vi "LocalisationFileLoader.vi"(11 "FilePath":path) -> (3 "LocalisationFileContent[out]":T1)   [LabVIEW 2012]
uses:
  <vilib>/Utility/file.llb/Read From Spreadsheet File (string).vi
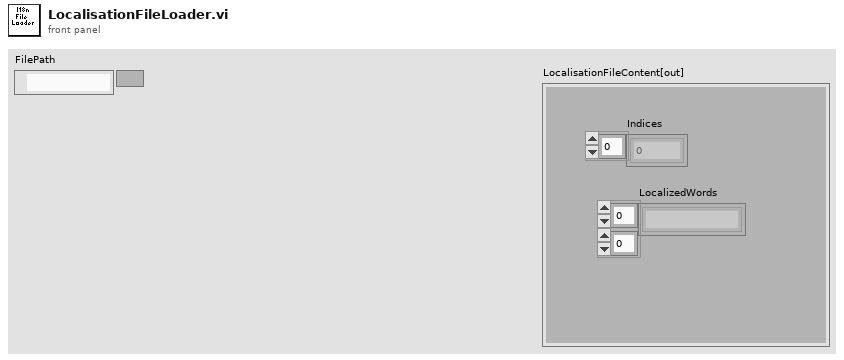
[diagram p1: front panel]
types:
  T1 = cluster{"Indices":u32[], "LocalizedWords":string[][]}
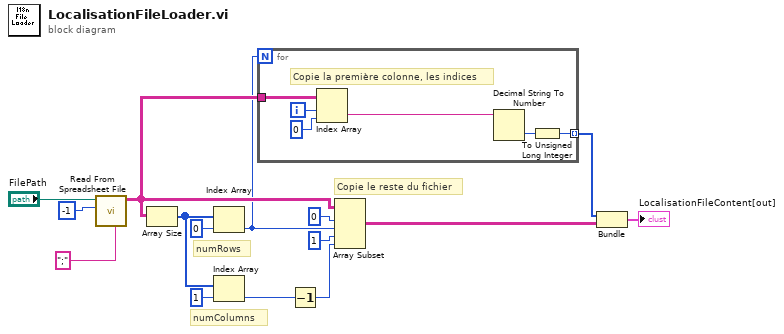
[diagram p0: block diagram]
diagram:
  # "Copie le reste du fichier"
  # "numColumns"
  # "numRows"
  n1 = call-poly <vilib>:"Read From Spreadsheet File.vi"("delimiter (\\t)"=";", "number of rows (all:-1)"=-1, "file path (dialog if empty)"="FilePath") -> ("all rows"=w8:string[][])  [unwired: 4 in, 4 out]
  n2 = Array Size(array=w8) -> (size(s)=w11:i32[])
  n3 = Index Array(array=w11, index=0) -> (element=w2:i32)
  n4 = Index Array(array=w11, index=1) -> (element=w4:i32)
  n5 = for {
    N: w2 -> [_]
    tunnel: w8 -> [w20]
    tunnel: [w16] -> w1 mode=indexing
    i -> [w21]
    # "Copie la première colonne, les indices"
    n6 = Index Array(array=w20, index (row)=w21, index (col)=0) -> (element=w19:string)
    n7 = Decimal String To Number(string=w19) -> (number=w17:i32)  [unwired: 2 in, 1 out]
    n8 = To Unsigned Long Integer(number=w17) -> (unsigned 32bit integer=w16:u32)
  }
  n9 = Decrement(x=w4) -> (x-1=w5:i32)
  n10 = Array Subset(array=w8, index (row)=0, length (row)=w2, index (col)=1, length (col)=w5) -> (w3:string[][])
  n11 = Bundle(w1, w3) -> (→"LocalisationFileContent[out]":cluster{u32[], string[][]})  [unwired: 1 in]
